vi "RB Helper Main.vi"() -> ()   [LabVIEW 2015]
uses:
  Cities Enum.ctl
  Regions Enum.ctl
panel:
  out "Destination":T1
  in  "Region":T2
  in  "Find New Destination":bool
  in  "Dest City":T1
  out "Payoff":dbl format="$%d"
  in  "Start City":T1
  # "Destination Finder"
  # "Payoff Calculator"
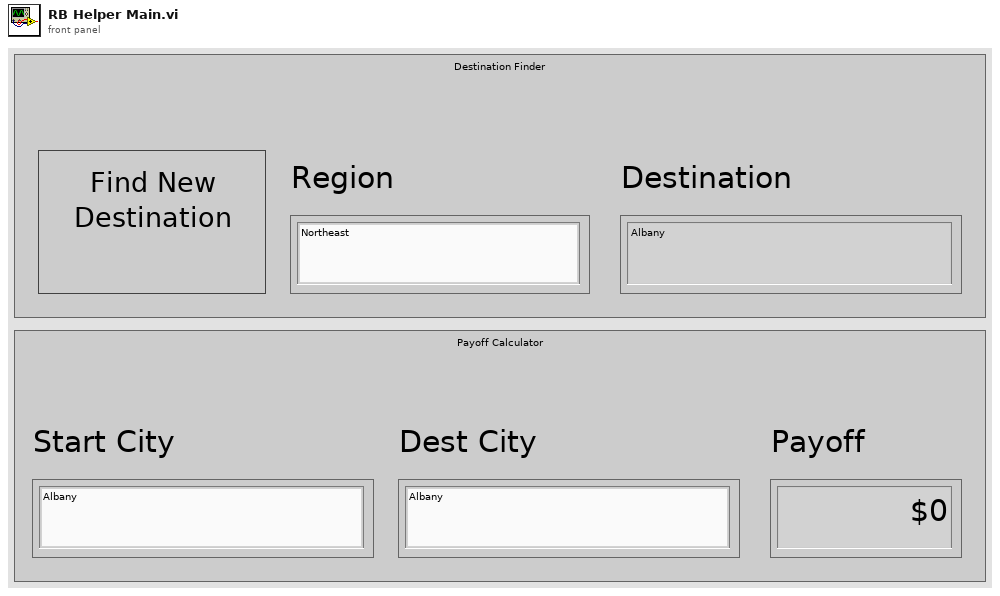
[diagram p1: front panel]
types:
  T1 = typedef "Cities Enum.ctl" = enum16{"Albany", "Baltimore", "Boston", "Buffalo", "New York", "Philadelphia", "Pittsburgh", "ME, Portland", "Washington", "Atlanta", "Charleston", "Charlotte", "Chattanooga", "Jacksonville", "Knoxville", "Miami", "Mobile", "Norfolk", "Richmond", "Tampa", "Chicago", "Cincinnati", "Cleveland", "Columbus", "Detroit", "Indianapolis", "Milwaukee", "StLouis", "Birmingham", "Dallas", "Fort Worth", "Houston", "Little Rock", "Louisville", "Memphis", "Nashville", "New Orleans", "San Antonio", "Shreveport", "Denver", "Des Moines", "Fargo", "Kansas City", "Minneapolis", "Oklahoma City", "Omaha", "Pueblo", "StPaul", "Billings", "Butte", "Casper", "Pocatello", "OR, Portland", "Rapid City", "Salt Lake City", "Seattle", "Spokane", "El Paso", "Las Vegas", "Los Angeles", "Oakland", "Phoenix", "Reno", "Sacramento", "San Diego", "San Francisco", "Tucumcari"}
  T2 = typedef "Regions Enum.ctl" = enum16{"Northeast", "Southeast", "North Central", "South Central", "Plains", "Northwest", "Southwest"}
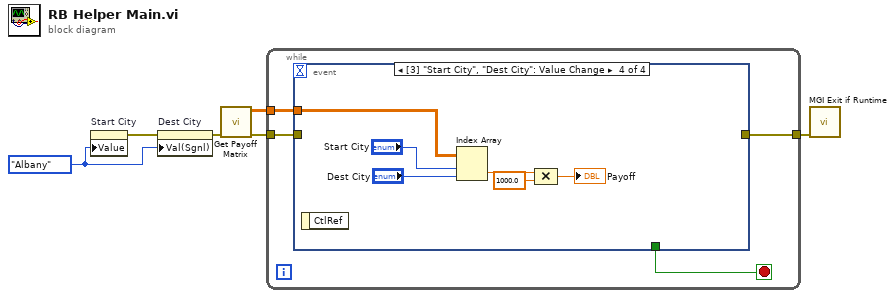
[diagram p0: block diagram]
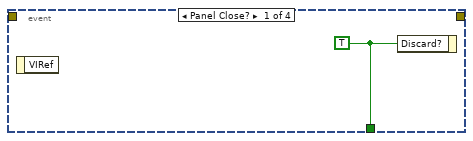
[diagram p2: hidden frame]
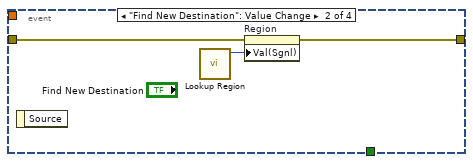
[diagram p3: hidden frame]
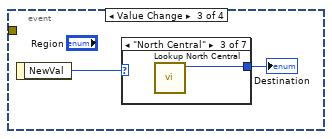
[diagram p4: hidden frame]
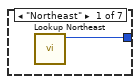
[diagram p5: hidden frame]
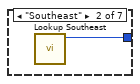
[diagram p6: hidden frame]
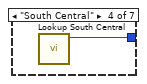
[diagram p7: hidden frame]
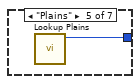
[diagram p8: hidden frame]
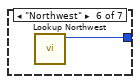
[diagram p9: hidden frame]
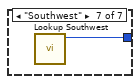
[diagram p10: hidden frame]
diagram:
  w3 = Cities_Enum."Albany" ("Start City")
  n1 = property on="Start City" class="Enum (strict)"("Value"=w3) -> (error out=w5:errorcluster)  [unwired: 2 in, 1 out]
  n2 = property on="Dest City" class="Enum (strict)"(error in=w5, "Val(Sgnl)"=w3) -> (error out=w4:errorcluster)  [unwired: 1 in, 1 out]
  n3 = call "Get Payoff Matrix.vi"("error in (no error)"=w4) -> ("error out"=w1:errorcluster, "Payoff Matrix"=w6:dbl[][])  [unwired: 9 in]
  n4 = while {
    tunnel: w6 -> [w9]
    tunnel: [w7] -> w2
    tunnel: w1 -> [w8]
    stop <- w10 stop-if-true
    n5 = event shown="[3] \"Start City\", \"Dest City\": Value Change" {
      selector: _ -> [_ _ _ _]
      dyn-events: _ -> [_ _ _ _]
      timeout: _ -> [_ _ _ _]
      tunnel: [w11 _ _ _] -> w10
      tunnel: w9 -> [_ _ _ w24]
      tunnel: w8 -> [_ w14 _ _]
      tunnel: [_ w12 _ _] -> w7
      event Panel Close? {
        w11 = TRUE ("Discard?")
        n6 = event-data() -> ()  [unwired: 1 in, 1 out]
        n7 = event-data("Discard?"=w11) -> ()  [unwired: 1 in, 1 out]
      }
      event "Find New Destination": Value Change {
        n8 = event-data() -> ()  [unwired: 1 in, 1 out]
        n9 = call "Lookup Region.vi"() -> ("Region"=w13:T2)  [unwired: 11 in]
        n10 = property on="Region" class="Enum (strict)"(error in=w14, "Val(Sgnl)"=w13) -> (error out=w12:errorcluster)  [unwired: 1 in, 1 out]
      }
      event Value Change {
        n11 = event-data() -> ("NewVal"=w16:T2)  [unwired: 1 in]
        n12 = case shown="\"North Central\"" w16 {
          tunnel: [w17 w18 w19 w20 w21 w22 w23] -> w15
          frame "Northeast" {
            n13 = call "Lookup Northeast.vi"() -> ("City"=w17:T1)  [unwired: 11 in]
          }
          frame "Southeast" {
            n14 = call "Lookup Southeast.vi"() -> ("City"=w18:T1)  [unwired: 11 in]
          }
          frame "North Central" {
            n15 = call "Lookup North Central.vi"() -> ("City"=w19:T1)  [unwired: 11 in]
          }
          frame "South Central" {
            n16 = call "Lookup South Central.vi"() -> ("City"=w20:T1)  [unwired: 11 in]
          }
          frame "Plains" {
            n17 = call "Lookup Plains.vi"() -> ("City"=w21:T1)  [unwired: 11 in]
          }
          frame "Northwest" {
            n18 = call "Lookup Northwest.vi"() -> ("City"=w22:T1)  [unwired: 11 in]
          }
          frame "Southwest" {
            n19 = call "Lookup Southwest.vi"() -> ("City"=w23:T1)  [unwired: 11 in]
          }
        }
        "Destination" <- w15
      }
      event Value Change {
        n20 = event-data() -> ()  [unwired: 1 in, 1 out]
        n21 = Index Array(array=w24, index (row)="Start City", index (col)="Dest City") -> (element=w27:dbl)
        n22 = Compound Arithmetic op=MULTIPLY(w27, 1000.0 ("value")) -> (→"Payoff":dbl)
      }
    }
  }
  n23 = call <userlib>:"MGI Exit if Runtime.vi"("Error In (Dependency Only)"=w2) -> ()  [unwired: 11 in]
